vi "proc_check_exit_code.vi"(8 "error in":errorcluster, 10 "ignore error":bool=TRUE, 11 "instance handle in":u32[](array[numeric])) -> (0 "error out":errorcluster, 1 "exited":bool, 2 "running":bool, 3 "instance handle out":u32[](array[numeric]), 4 "exit code":i32)   [LabVIEW 2011]
doc: "This VI checks process instance status. It signalizes if Octave is still running or already returned exit code. In that case exit code it returned.\nIf no process instance handle is connected, last one from global variable is used or new instance handle is stored to it.\nProcess instance handle can be automatically closed if process has exited."
panel:
  in  "exit code buf":i32
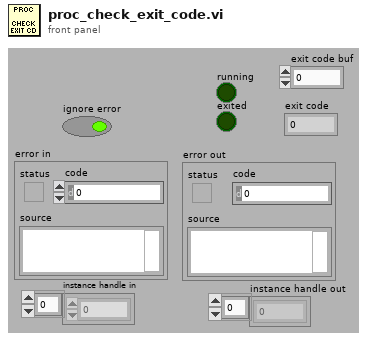
[diagram p1: front panel]
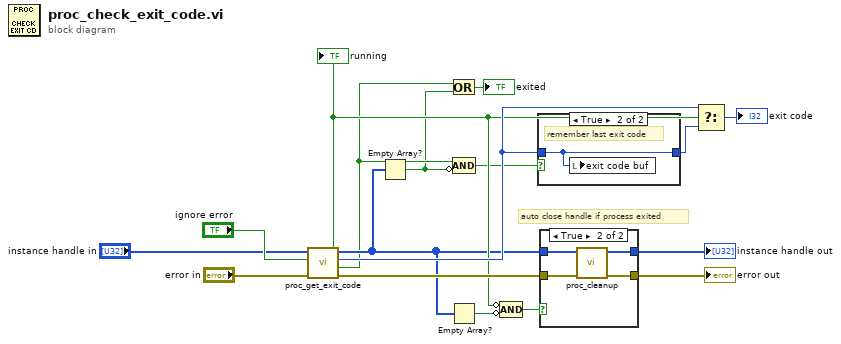
[diagram p0: block diagram]
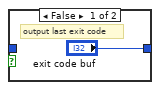
[diagram p2: hidden frame]
diagram:
  # "auto close handle if process exited"
  n1 = call "proc_get_exit_code.vi"("error in"="error in", "ignore error"="ignore error", "process instance handle in"="instance handle in") -> ("error out"=w9:errorcluster, "exited"=w2:bool, "exit code"=w8:i32, "process instance handle out"=w4:u32[], "running"=w7:bool)  [unwired: 4 in]
  "running" <- w7
  n2 = Empty Array?(array=w4) -> (empty?=w1:bool)
  n3 = Or(x=w2, y=w1) -> (x .or. y?=→"exited":bool)
  n4 = Empty Array?(array=w4) -> (empty?=w14:bool)
  n5 = Compound Arithmetic op=AND(w2, invert w1) -> (w6:bool)
  n6 = Compound Arithmetic op=AND(invert w7, invert w14) -> (w15:bool)
  n7 = case shown="True" w6 {
    tunnel: w8 -> [_ w19]
    tunnel: ["exit code buf" w19] -> w13
    frame False {
      # "output last exit code"
    }
    frame True {
      # "remember last exit code"
      n8 = local write "exit code buf"(w19) -> ()
    }
  }
  n9 = case shown="True" w15 {
    tunnel: w9 -> [w20 w25]
    tunnel: [w20 w24] -> w11
    tunnel: [w21 w23] -> w12
    tunnel: w4 -> [w21 w22]
    frame False {
    }
    frame True {
      n10 = call "proc_cleanup.vi"("error in"=w25, "process instance handle in"=w22) -> ("error out"=w24:errorcluster, "process instance handle out"=w23:u32[])  [unwired: 8 in]
    }
  }
  "error out" <- w11
  "instance handle out" <- w12
  n11 = Select(t=w8, s=w7, f=w13) -> (s? t:f=→"exit code":i32)
